vi "Lithographify_funnel&rec.vi"(5 "Data In":cluster{string, cluster{"X":dbl, "Y":dbl}[]}, 7 "Direction":u16, 9 "Speed (µm/s)":T1={"Schedule"=0, "Value"=0.0, "Start Value"=0.0, "End Value"=0.0, "Min Value"=0.0, "Max Value"=0.0, "Duty Cycle (%)"=0.0, "Signal Type"=0, "Cycle Number"=0.0, "Phase (degrees)"=0.0, "formula"="1*(step(170-t)*cos(0.62831853071*t)+step(t-170)*cos(0.62831853071*(t-170))*(-1))", "formula length (nm)"=340.0, "formula resolution (nm)"=0.001} {"Signal Type" items=["Sine Wave", "Triangle Wave", "Square Wave", "Sawtooth Wave"]; "Schedule" items=["Constant", "Ramp", "Fn. Generator", "Formula"]}, 11 "Voltage (V)":T1={"Schedule"=0, "Value"=0.0, "Start Value"=0.0, "End Value"=0.0, "Min Value"=0.0, "Max Value"=0.0, "Duty Cycle (%)"=0.0, "Signal Type"=0, "Cycle Number"=0.0, "Phase (degrees)"=0.0, "formula"="1*(step(170-t)*cos(0.62831853071*t)+step(t-170)*cos(0.62831853071*(t-170))*(-1))", "formula length (nm)"=340.0, "formula resolution (nm)"=0.001} {"Signal Type" items=["Sine Wave", "Triangle Wave", "Square Wave", "Sawtooth Wave"]; "Schedule" items=["Constant", "Ramp", "Fn. Generator", "Formula"]}, 13 "Enabled":bool) -> (4 "Lithography Data":T4)   [LabVIEW 2016]
doc: "This VI calculates the lithography data of one pattern and organizes it appropriately."
uses:
  typedefs/Voltage - cluster.ctl
  typedefs/Schedule - enum.ctl
  typedefs/Signal Type - enum.ctl
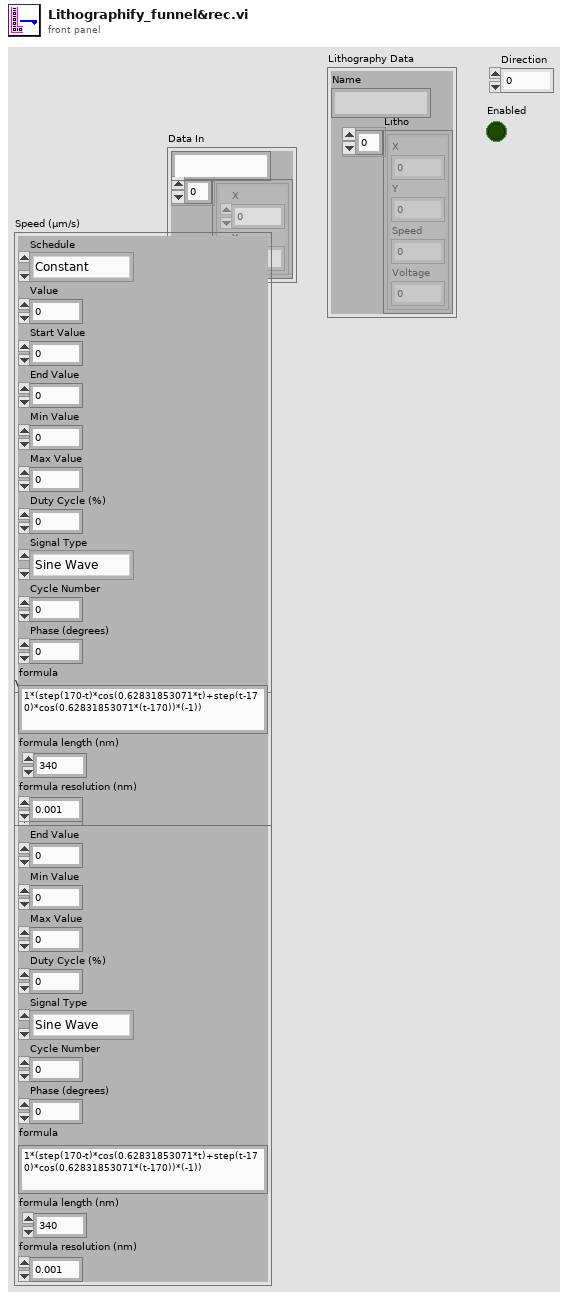
[diagram p1: front panel]
types:
  T1 = typedef "Voltage - cluster.ctl" = cluster{"Schedule":T2, "Value":dbl, "Start Value":dbl, "End Value":dbl, "Min Value":dbl, "Max Value":dbl, "Duty Cycle (%)":dbl, "Signal Type":T3, "Cycle Number":dbl, "Phase (degrees)":dbl, "formula":string, "formula length (nm)":dbl, "formula resolution (nm)":dbl}
  T2 = typedef "Schedule - enum.ctl" = u16
  T3 = typedef "Signal Type - enum.ctl" = u16
  T4 = cluster{"Name":string, "Litho":cluster{"X":dbl, "Y":dbl, "Speed":dbl, "Voltage":dbl}[]}
  T5 = cluster{"X":dbl, "Y":dbl, "Speed":dbl, "Voltage":dbl}[]
  T6 = cluster{"X":dbl, "Y":dbl, "Speed":dbl, "Voltage":dbl}
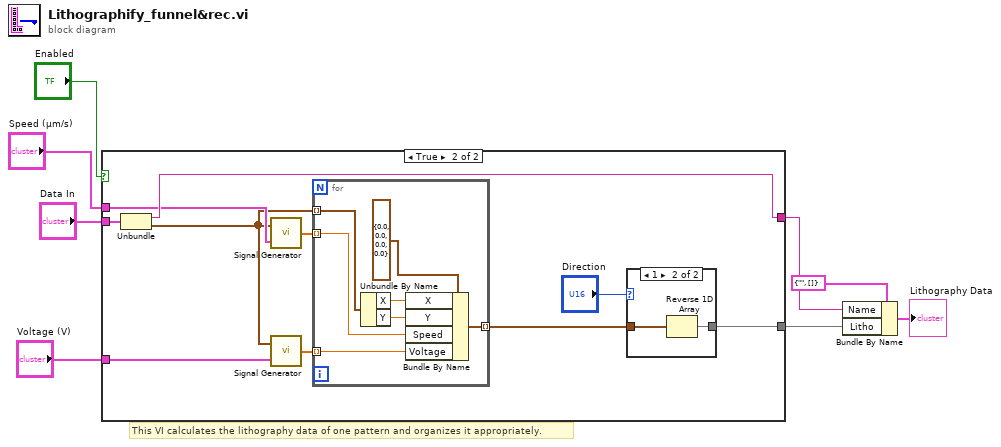
[diagram p0: block diagram]
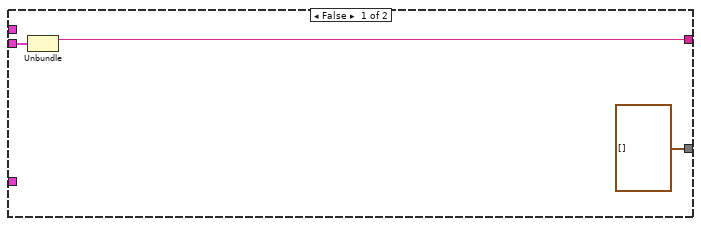
[diagram p2: hidden frame]
diagram:
  # "This VI calculates the lithography data of one pattern and organizes it appropriately."
  n1 = case shown="True" "Enabled" {
    tunnel: [w10 w21] -> w8
    tunnel: "Data In" -> [w11 w20]
    tunnel: "Voltage (V)" -> [_ w17]
    tunnel: "Speed (µm/s)" -> [_ w16]
    tunnel: [T5 [] w14] -> w2
    frame False {
      n2 = Unbundle(w11) -> (w10:string)  [unwired: 1 out]
    }
    frame True {
      n3 = Unbundle(w20) -> (w21:string, w12:cluster{"X":dbl, "Y":dbl}[])
      n4 = call "Signal Generator.vi"("Signal Properties"=w16, "Points"=w12) -> ("Signal"=w18:dbl[])
      n5 = call "Signal Generator.vi"("Signal Properties"=w17, "Points"=w12) -> ("Signal"=w19:dbl[])
      n6 = for {
        tunnel: w18 -> [w27] mode=indexing
        tunnel: w19 -> [w26] mode=indexing
        tunnel: w12 -> [w29] mode=indexing
        tunnel: [w25] -> w15 mode=indexing
        n7 = Unbundle By Name(w29) -> ("X"=w30:dbl, "Y"=w28:dbl)
        n8 = Bundle By Name(cluster=T6 {"X"=0.0, "Y"=0.0, "Speed"=0.0, "Voltage"=0.0} ("Litho Point"), "X"=w30, "Y"=w28, "Speed"=w27, "Voltage"=w26) -> (w25:T6)
      }
      n9 = case shown="1" "Direction" {
        tunnel: w15 -> [w22 w24]
        tunnel: [w22 w23] -> w14
        frame 0, Default {
        }
        frame 1 {
          n10 = Reverse 1D Array(array=w24) -> (reversed array=w23:T5)
        }
      }
    }
  }
  n11 = Bundle By Name(cluster=T4 {"Name"="", "Litho"=[]} ("Lithography Data"), "Name"=w8, "Litho"=w2) -> (→"Lithography Data":T4)
